vi "Make Details File.vi"(4 "Duty cycle (%)":dbl, 5 "Comments":string, 6 "Number of samples per s":dbl, 7 "Frequency":dbl, 9 "405 LED Power":dbl, 10 "470 LED power":dbl, 11 "created path":path) -> ()   [LabVIEW 2018]
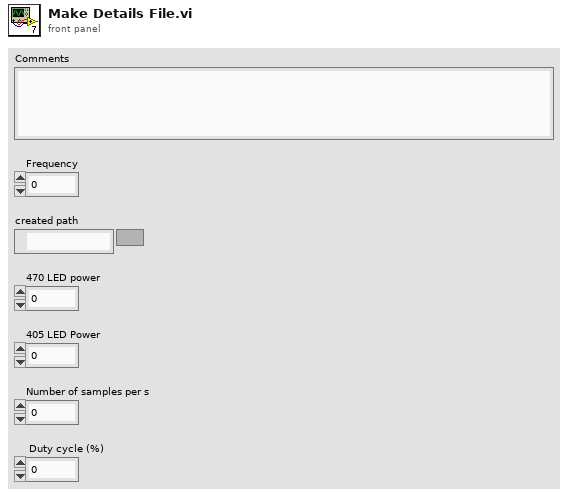
[diagram p1: front panel]
types:
  T1 = enum16{"open", "replace", "create", "open or create", "replace or create", "replace or create with confirmation"}
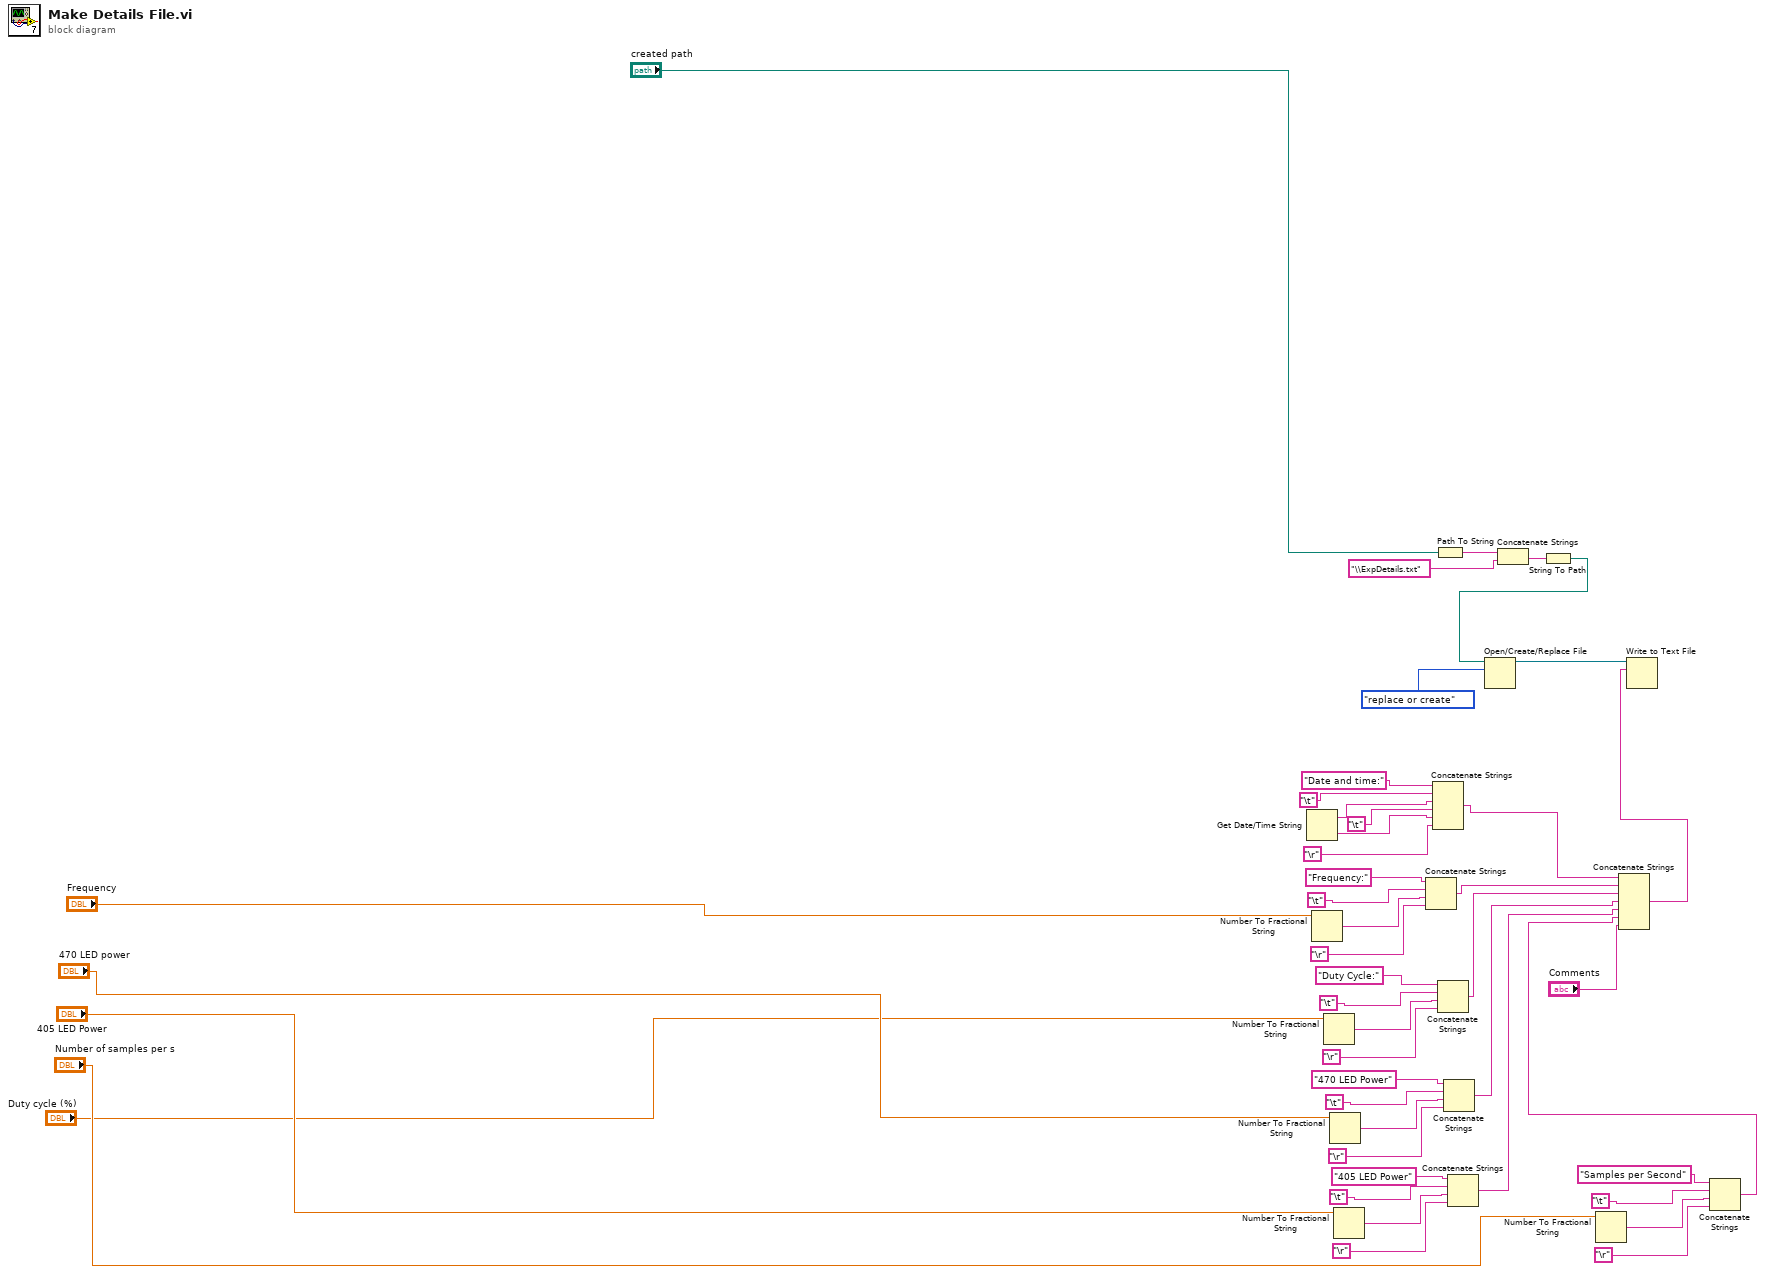
[diagram p0: block diagram]
diagram:
  n1 = Get Date/Time String() -> (date string=w5:string, time string=w7:string)  [unwired: 3 in]
  n2 = Number To Fractional String(number="Frequency") -> (F-format string=w12:string)  [unwired: 3 in]
  n3 = Number To Fractional String(number="Duty cycle (%)") -> (F-format string=w14:string)  [unwired: 3 in]
  n4 = Number To Fractional String(number="470 LED power") -> (F-format string=w19:string)  [unwired: 3 in]
  n5 = Number To Fractional String(number="405 LED Power") -> (F-format string=w22:string)  [unwired: 3 in]
  n6 = Concatenate Strings("Frequency:", "\t", w12, "\r") -> (w35:string)
  n7 = Concatenate Strings("Date and time:", "\t", w5, "\t", w7, "\r") -> (w34:string)
  n8 = Path To String(path="created path") -> (string=w42:string)
  n9 = Concatenate Strings("Duty Cycle:", "\t", w14, "\r") -> (w36:string)
  n10 = Concatenate Strings("470 LED Power", "\t", w19, "\r") -> (w37:string)
  n11 = Concatenate Strings("405 LED Power", "\t", w22, "\r") -> (w38:string)
  n12 = Concatenate Strings(w42, "\\ExpDetails.txt") -> (w44:string)
  n13 = String To Path(string=w44) -> (path=w45:path)
  n14 = Open/Create/Replace File(file path (use dialog)=w45, operation (0:open)=T1."replace or create") -> (refnum out=w2:refnum<file>)  [unwired: 4 in, 2 out]
  n15 = Number To Fractional String(number="Number of samples per s") -> (F-format string=w25:string)  [unwired: 3 in]
  n16 = Concatenate Strings("Samples per Second", "\t", w25, "\r") -> (w39:string)
  n17 = Concatenate Strings(w34, w35, w36, w37, w38, w39, "Comments") -> (w40:string)
  n18 = Write to Text File(file (use dialog)=w2, text=w40) -> ()  [unwired: 2 in, 3 out]
